vi "Scripting Replace Message.vi"(8 "error in":errorcluster, 10 "New Message":string, 11 "Path":path) -> (0 "error out":errorcluster)   [LabVIEW 2026]
uses:
  <vilib>/Utility/traverseref.llb/TRef TravTarget.ctl
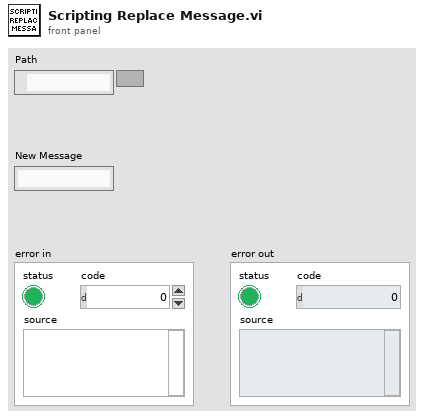
[diagram p1: front panel]
types:
  T1 = typedef "TRef TravTarget.ctl" = enum16{"FP", "BD", "Other"}
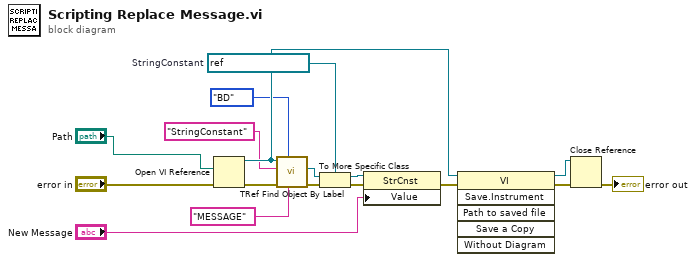
[diagram p0: block diagram]
diagram:
  w8 = refnum<vi> refnum  # StringConstant
  n1 = Open VI Reference(vi path="Path", error in (no error)="error in") -> (vi reference=w5:refnum<vi>, error out=w16:errorcluster)  [unwired: 4 in]
  n2 = call <vilib>:"TRef Find Object By Label.vi"("Label"="MESSAGE" ("Class Name"), "Traverse Target"=TRef_TravTarget."BD", "error in (no error)"=w16, "Class Name"="StringConstant", "VI Ref"=w5) -> ("error out"=w15:errorcluster, "Found Obj Ref"=w9:refnum<vi>)  [unwired: 3 in, 2 out]
  n3 = To More Specific Class(target class=w8, reference=w9, error in=w15) -> (specific class reference=w7:refnum<vi>, error out=w14:errorcluster)
  n4 = property class="StrCnst"(reference=w7, error in=w14, "Value"="New Message") -> (error out=w13:errorcluster)  [unwired: 1 out]
  n5 = invoke class="VI" method="Save.Instrument"(reference=w5, error in=w13) -> (reference out=w4:refnum<vi>, error out=w12:errorcluster)  [unwired: 4 in, 4 out]
  n6 = Close Reference(reference=w4, error in (no error)=w12) -> (error out=→"error out":errorcluster)
